vi "ThreadCfg - Write RxPkt Config.vi"(8 "error in (no error)":errorcluster, 10 "threadOptions":T1 {"pclDecimation" max=16 step=1; "loopPeriod" min=-2 max=16 step=1; "targetPriority" min=-2 max=16 step=1; "targetProcessor" min=-2 max=16 step=1}, 11 "Node Ptr In":T3 format="%.0x") -> (0 "error out":errorcluster, 3 "Node Ptr Out":T3 format="%.0x")   [LabVIEW 2016, in "UDP-Custom-Device System Explorer.lvlib"]
uses:
  UDP-Custom-Device System Explorer.lvlib
  <vilib>/NI Veristand/Custom Device API/Custom Device Item Ref.ctl
  Types/Threading/Thread Configuration.ctl
  Types/Threading/Thread Sync Reference.ctl
  Property Accessors/Shared Packet Accessors.lvlib
  <vilib>/NI VeriStand/Custom Device API/Custom Device API.lvlib
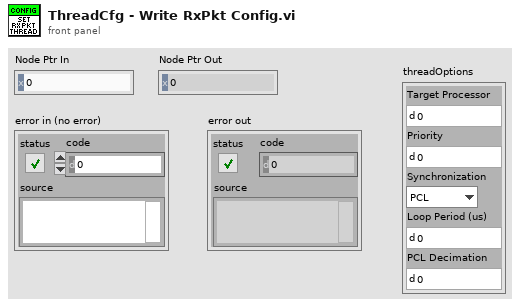
[diagram p1: front panel]
types:
  T1 = typedef "UDP-Custom-Device System Explorer.lvlib/Thread Configuration.ctl" = cluster{"targetProcessor":i8, "targetPriority":i16, "Synchronization":T2, "loopPeriod":i32, "pclDecimation":u16}
  T2 = typedef "UDP-Custom-Device System Explorer.lvlib/Thread Sync Reference.ctl" = enum16{"PCL", "Async"}
  T3 = typedef "Custom Device API.lvlib/Custom Device Item Ref.ctl" = u64
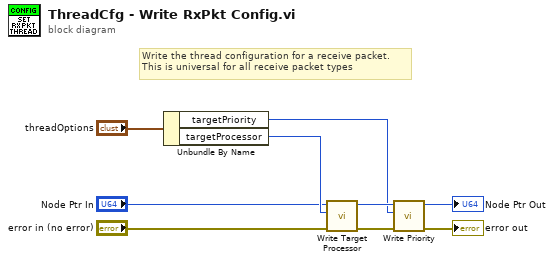
[diagram p0: block diagram]
diagram:
  # "Write the thread configuration for a receive packet.\nThis is universal for all receive packet types"
  n1 = Unbundle By Name("threadOptions") -> ("targetPriority"=w3:i16, "targetProcessor"=w4:i8)
  n2 = call "Write Target Processor.vi"("error in (no error)"="error in (no error)", "targetProcessor"=w4, "Node Ptr"="Node Ptr In") -> ("error out"=w9:errorcluster, "Node Ptr out"=w5:T3)  [unwired: 7 in]
  n3 = call "Write Priority.vi"("error in (no error)"=w9, "targetPriority"=w3, "Node Ptr"=w5) -> ("error out"=→"error out":errorcluster, "Node Ptr out"=→"Node Ptr Out":T3)  [unwired: 7 in]
